vi "load_S_curve.vi"(10 "samples":i32=2500000, 11 "pulses":i32=500) -> (2 "Raw S Curve":u32[](graph), 3 "S Curve":u32[](graph))   [LabVIEW 2017]
panel:
  out "sum":i32
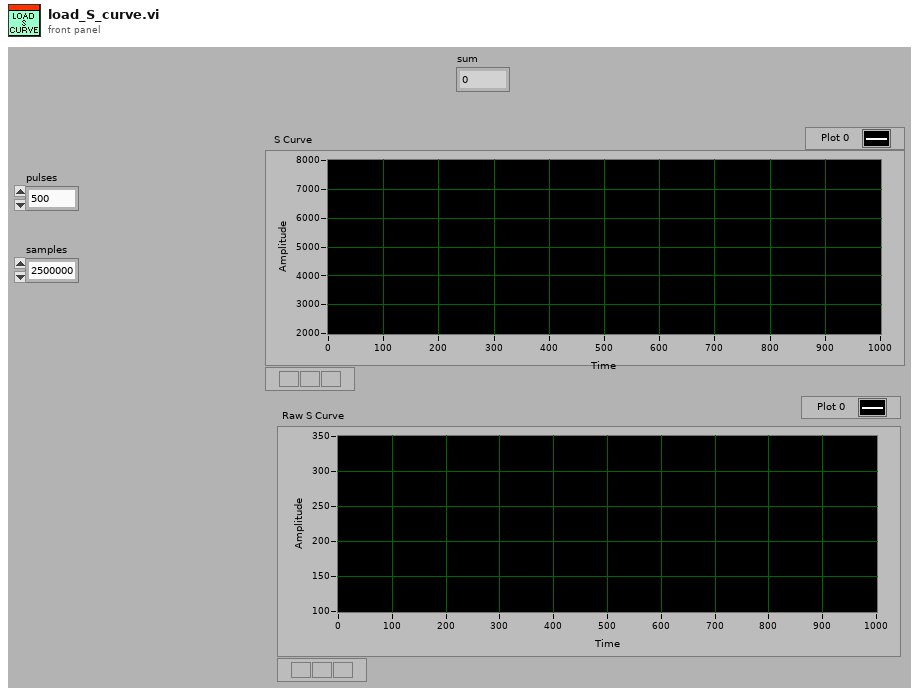
[diagram p1: front panel]
types:
  T1 = enum16{"big-endian, network order", "native, host order", "little-endian"}
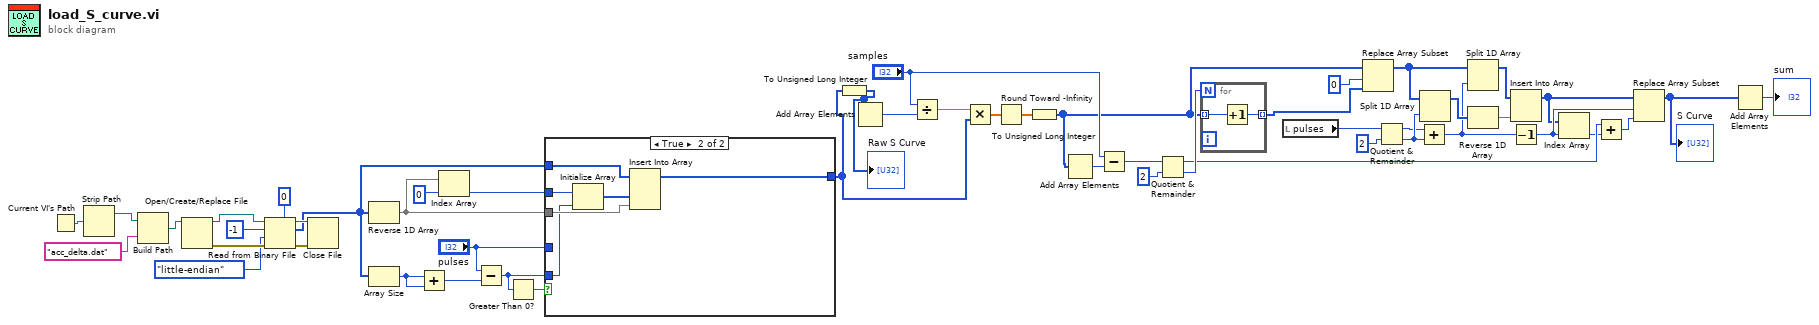
[diagram p0: block diagram]
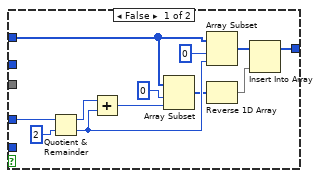
[diagram p2: hidden frame]
diagram:
  n1 = Current VI's Path() -> (path=w4:path)
  n2 = Strip Path(path=w4) -> (stripped path=w3:path)  [unwired: 1 out]
  n3 = Build Path(base path=w3, name or relative path="acc_delta.dat") -> (appended path=w1:path)
  n4 = Open/Create/Replace File(file path (use dialog)=w1) -> (refnum out=w49:refnum<file>, error out=w50:errorcluster)  [unwired: 5 in, 1 out]
  n5 = Read from Binary File(5:i16 0, 8:w50, 9:T1."little-endian" ("byte order (0:big-endian, network order)"), 10:-1 ("count (1)"), 11:w49) -> (0:w46:errorcluster, 2:w10:i16[], 3:w47:refnum<file>)  [unwired: 1 in, 1 out]
  n6 = Close File(refnum=w47, error in=w46) -> ()  [unwired: 2 out]
  n7 = Reverse 1D Array(array=w10) -> (reversed array=w41:i16[])
  n8 = Array Size(array=w10) -> (size(s)=w45:i32)
  n9 = Add(x=w45, y=w45) -> (x+y=w44:i32)
  n10 = Index Array(array=w41, index=0) -> (element=w42:i16)
  n11 = Subtract(x="pulses", y=w44) -> (x-y=w33:i32)
  n12 = Greater Than 0?(x=w33) -> (x > 0?=w32:bool)
  n13 = case shown="True" w32 {
    tunnel: w42 -> [_ w68]
    tunnel: w10 -> [w58 w67]
    tunnel: w41 -> [_ w65]
    tunnel: [w51 w64] -> w9
    tunnel: w33 -> [_ w63]
    tunnel: "pulses" -> [w61 _]
    frame False {
      n14 = Quotient & Remainder(x=w61, y=2) -> (x-y*floor(x/y)=w57:i32, floor(x/y)=w56:i32)
      n15 = Add(x=w57, y=w56) -> (x+y=w55:i32)
      n16 = Array Subset(array=w58, index=0, length=w55) -> (w54:i16[])
      n17 = Array Subset(array=w58, index=0, length=w56) -> (w53:i16[])
      n18 = Reverse 1D Array(array=w54) -> (reversed array=w52:i16[])
      n19 = Insert Into Array(array=w53, new element=w52) -> (w51:i16[])  [unwired: 1 in]
    }
    frame True {
      n20 = Initialize Array(w68, w63) -> (w66:i16[])
      n21 = Insert Into Array(array=w67, new element #1=w66, new element #2=w65) -> (w64:i16[])  [unwired: 1 in]
    }
  }
  n22 = To Unsigned Long Integer(number=w9) -> (unsigned 32bit integer=w7:u32[])
  "Raw S Curve" <- w7
  n23 = Add Array Elements(numeric array=w7) -> (sum=w8:u32)
  n24 = Divide(x="samples", y=w8) -> (x/y=w38:dbl)
  n25 = Multiply(x=w38, y=w9) -> (x*y=w37:dbl[])
  n26 = Round Toward -Infinity(1:w37) -> (0:w36:dbl[])
  n27 = To Unsigned Long Integer(number=w36) -> (unsigned 32bit integer=w6:u32[])
  n28 = Add Array Elements(numeric array=w6) -> (sum=w39:u32)
  n29 = Subtract(x="samples", y=w39) -> (x-y=w31:u32)
  n30 = Quotient & Remainder(x=w31, y=2) -> (x-y*floor(x/y)=w27:u32, floor(x/y)=w29:u32)
  n31 = for {
    N: w29 -> [_]
    tunnel: w6 -> [w70] mode=indexing
    tunnel: [w69] -> w34 mode=indexing
    n32 = Increment(x=w70) -> (x+1=w69:u32)
  }
  n33 = local read "pulses"() -> (w13:i32)
  n34 = Replace Array Subset(array=w6, new element=w34, index=0) -> (w16:u32[])
  n35 = Quotient & Remainder(x=w13, y=2) -> (x-y*floor(x/y)=w19:i32, floor(x/y)=w20:i32)
  n36 = Add(x=w19, y=w20) -> (x+y=w18:i32)
  n37 = Split 1D Array(array=w16, index=w20) -> (first subarray=w24:u32[])  [unwired: 1 out]
  n38 = Split 1D Array(array=w16, index=w18) -> (first subarray=w23:u32[])  [unwired: 1 out]
  n39 = Reverse 1D Array(array=w24) -> (reversed array=w22:u32[])
  n40 = Insert Into Array(array=w23, new element=w22) -> (w15:u32[])  [unwired: 1 in]
  n41 = Decrement(x=w18) -> (x-1=w17:i32)
  n42 = Index Array(array=w15, index=w17) -> (element=w26:u32)
  n43 = Add(x=w27, y=w26) -> (x+y=w25:u32)
  n44 = Replace Array Subset(array=w15, new element=w25, index=w17) -> (w5:u32[])
  "S Curve" <- w5
  n45 = Add Array Elements(numeric array=w5) -> (sum=→"sum":u32)
